vi "SLSC SPI Engine with CS.vi"(8 "error in (no error)":errorcluster, 9 "CS Bits":T1={"CS Bit 1"="Connector0/DIO0", "CS Bit 2"="Connector0/DIO0", "CS Bit 3"="Connector0/DIO0", "CS Bit 4"="Connector0/DIO0"}, 10 "SPI API References":T3, 11 "Chip Select DIO Lines":T2={"SCLK"="Port0/DIO3", "MISO"="Port0/DIO3", "MOSI"="Port0/DIO3", "CS 0"="Port0/DIO3", "CS 1"="Port0/DIO4", "CS 2"="Port0/DIO4", "CS 3"="Port0/DIO1", "CS 4"="Port0/DIO4", "CS 5"="Port0/DIO4"}) -> ()   [LabVIEW 2014, in "SLSC FPGA Toolkit.lvlib"]
uses:
  SLSC FPGA Toolkit.lvlib
  <vilib>/Platform/TimedLoop/XDataNode/wakeup.ctl
  <vilib>/Platform/TimedLoop/XDataNode/XDNodeRunTimeDep.lvlib
  <vilib>/Platform/TimedLoop/XDataNode/nitl_modes.ctl
  <vilib>/Platform/TimedLoop/XDataNode/timing_clust.ctl
  <vilib>/Platform/TimedLoop/XDataNode/XDataNode.xnode
  <vilib>/rvi/DataTransferAndStorage/Container/XNode/niFpgaContainer.xnode
  <vilib>/rvi/DataTransferAndStorage/Register/Emulation/niFpgaRegisterEmulation.vi
  <vilib>/SPI API/SPIAPI/Controls/Internal Data (SPI API).ctl
  <vilib>/SPI API/SPIAPI/DIO/SPI Digital IO Lines.ctl
  Source/Shared/SPI Utility/CS Bits.ctl
  Source/Shared/SLSC configuration Shared.lvlib
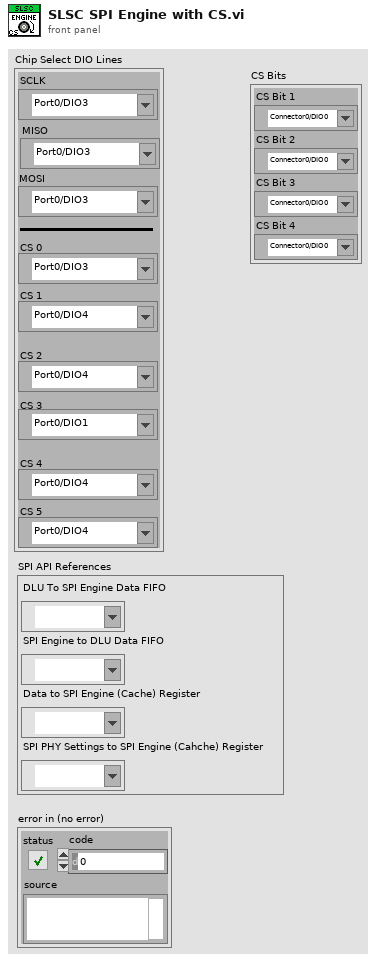
[diagram p1: front panel]
types:
  T1 = typedef "SLSC configuration Shared.lvlib/CS Bits.ctl" = cluster{"CS Bit 1":refnum<k21>, "CS Bit 2":refnum<k21>, "CS Bit 3":refnum<k21>, "CS Bit 4":refnum<k21>}
  T2 = typedef "SPI Digital IO Lines.ctl" = cluster{"SCLK":refnum<k21>, "MISO":refnum<k21>, "MOSI":refnum<k21>, "CS 0":refnum<k21>, "CS 1":refnum<k21>, "CS 2":refnum<k21>, "CS 3":refnum<k21>, "CS 4":refnum<k21>, "CS 5":refnum<k21>}
  T3 = typedef "Internal Data (SPI API).ctl" = cluster{"DLU To SPI Engine Data FIFO":refnum<k21>, "SPI Engine to DLU Data FIFO":refnum<k21>, "Data to SPI Engine (Cache) Register":refnum<k21>, "SPI PHY Settings to SPI Engine (Cahche) Register":refnum<k21>}
  T4 = typedef "XDNodeRunTimeDep.lvlib/timing_clust.ctl" = cluster{"Expected End [f-1]":u64, "Actual End [f-1]":u64, "Finished Late? [f-1]":bool, "Expected End [i-1]":u64, "Actual End [i-1]":u64, "Finished Late? [i-1]":bool, "Expected Start [i]":u64, "Actual Start [i]":u64, "Expected Start [f]":u64, "Actual Start [f]":u64, "Source Name":string, "Structure Name":string, "Period":i64, "Deadline":i64, "Offset":i64, "Start":i64, "Priority":i32, "Timeout":i32, "Mode":T5, "Wakeup Reason":T6, "Error":errorcluster, "Source Type":string, "Secondary Source Type":string, "Global End Time":u64, "Global Start Time":u64, "Frame Duration":u64, "Iteration Duration":u64, "Assigned CPU":i32, "I/O Scan Engine Mode":u32}
  T5 = typedef "XDNodeRunTimeDep.lvlib/nitl_modes.ctl" = enum32{"No Change", "Process missed periods, maintain original phase", "Discard missed periods, maintain original phase", "Process missed periods, ignore original phase", "Discard missed periods, ignore original phase"}
  T6 = typedef "XDNodeRunTimeDep.lvlib/wakeup.ctl" = enum32{"Normal", "Aborted", "Asynchronous wakeup", "Timing source error", "Timed loop error", "Timeout"}
  T7 = typedef "NI SPI IP FPGA.lvlib/Spi Master Inputs.ctl" = cluster{"MISO":bool}
  T8 = typedef "NI SPI IP FPGA.lvlib/Spi Master Outputs.ctl" = cluster{"Chip Select":bool, "Clock":bool, "MOSI":bool, "MOSI OE":bool}
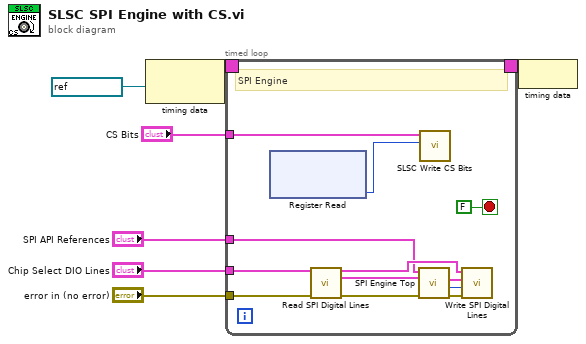
[diagram p0: block diagram]
diagram:
  n1 = node-c288(refnum<k21> "120MHz" ("Source Name")) -> (w7:T4)
  n2 = timed-loop {
    tunnel: "SPI API References" -> [w16]
    tunnel: "error in (no error)" -> [w14]
    tunnel: "Chip Select DIO Lines" -> [w18]
    timing: w7 -> [_]
    timing-out: [_] -> w6
    tunnel: "CS Bits" -> [w9]
    stop <- FALSE stop-if-true
    # "SPI Engine"
    n3 = xnode ("Register Read")() -> ("Data"=w8:u8)  [unwired: 1 in, 1 out]
    n4 = call <vilib>:"Read SPI Digital Lines.vi"("Chip Select DIO Lines"=w18, "error in"=w14) -> ("Chip Select DIO Lines Out"=w19:T2, "SPI Read Data"=w15:T7, "error out"=w13:errorcluster)  [unwired: 11 in]
    n5 = call <vilib>:"SPI Engine Top.vi"("error in"=w13, "SPI Read Data"=w15, "SPI API References"=w16) -> ("error out"=w12:errorcluster, "Chip Select ID"=w11:u8, "SPI DIO Output"=w17:T8)  [unwired: 5 in, 1 out]
    n6 = call "SLSC Write CS Bits.vi"("CS Bit Value/Slot #"=w8, "CS Bits"=w9) -> ()  [unwired: 10 in]
    n7 = call <vilib>:"Write SPI Digital Lines.vi"("error in"=w12, "CS Index"=w11, "spi output"=w17, "Chip Select DIO Lines"=w19) -> ()  [unwired: 6 in, 2 out]
  }
  n8 = node-c288(w6) -> ()
